vi "BN_outputLayer_with_FPGA.vi"(0 "Target_outX":fxp<+/-,32,8>[](array[numeric]), 1 "Out_hx":fxp<+/-,32,8>[](array[numeric]), 2 "Out_outX":fxp<+/-,32,8>[](array[numeric]), 3 "Learning rate":fxp<+/-,32,8>, 4 "Weights_outX_IN":fxp<+/-,32,8>[][](array[numeric])) -> (5 "Weights_outX_OUT":fxp<+/-,32,8>[][](array[numeric]))   [LabVIEW 2016]
uses:
  <vilib>/FPGAPlugInAG/myRIO-1900/niLvFpga_Open_myRIO-1900.vi
  <vilib>/rvi/interface/common/dynamic/niFpgaDynamicAddResources.vi
  <vilib>/Utility/error.llb/Error Cluster From Error Code.vi
  <vilib>/rvi/errors/niLvFpgaAdjustHostInterfaceError.vi
  <vilib>/FPGAPlugInAG/Dynamic/niLvFpga_Close_Dynamic.vi
  <vilib>/rvi/interface/nirviOpenFPGA/nirviOpenFPGA.xnode
  FPGA Bitfiles/Musicidentifier_FPGATarget_Update2layerWxFP_dcVOeM+zR40.lvbitx
  <vilib>/rvi/interface/nirviReadWriteControl/nirviReadWriteControl.xnode
  <vilib>/rvi/interface/nirviCloseFPGA/nirviCloseFPGA.xnode
  NiFpgaLv.dll
  <vilib>/rvi/interface/Simulation/niFpgaSimulationCallBeginRW.vi
panel:
  out "error out":errorcluster
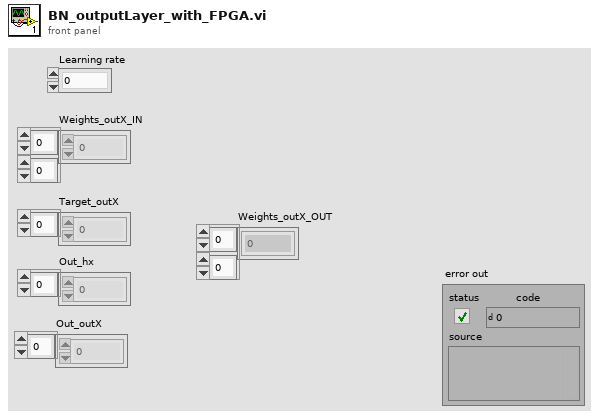
[diagram p1: front panel]
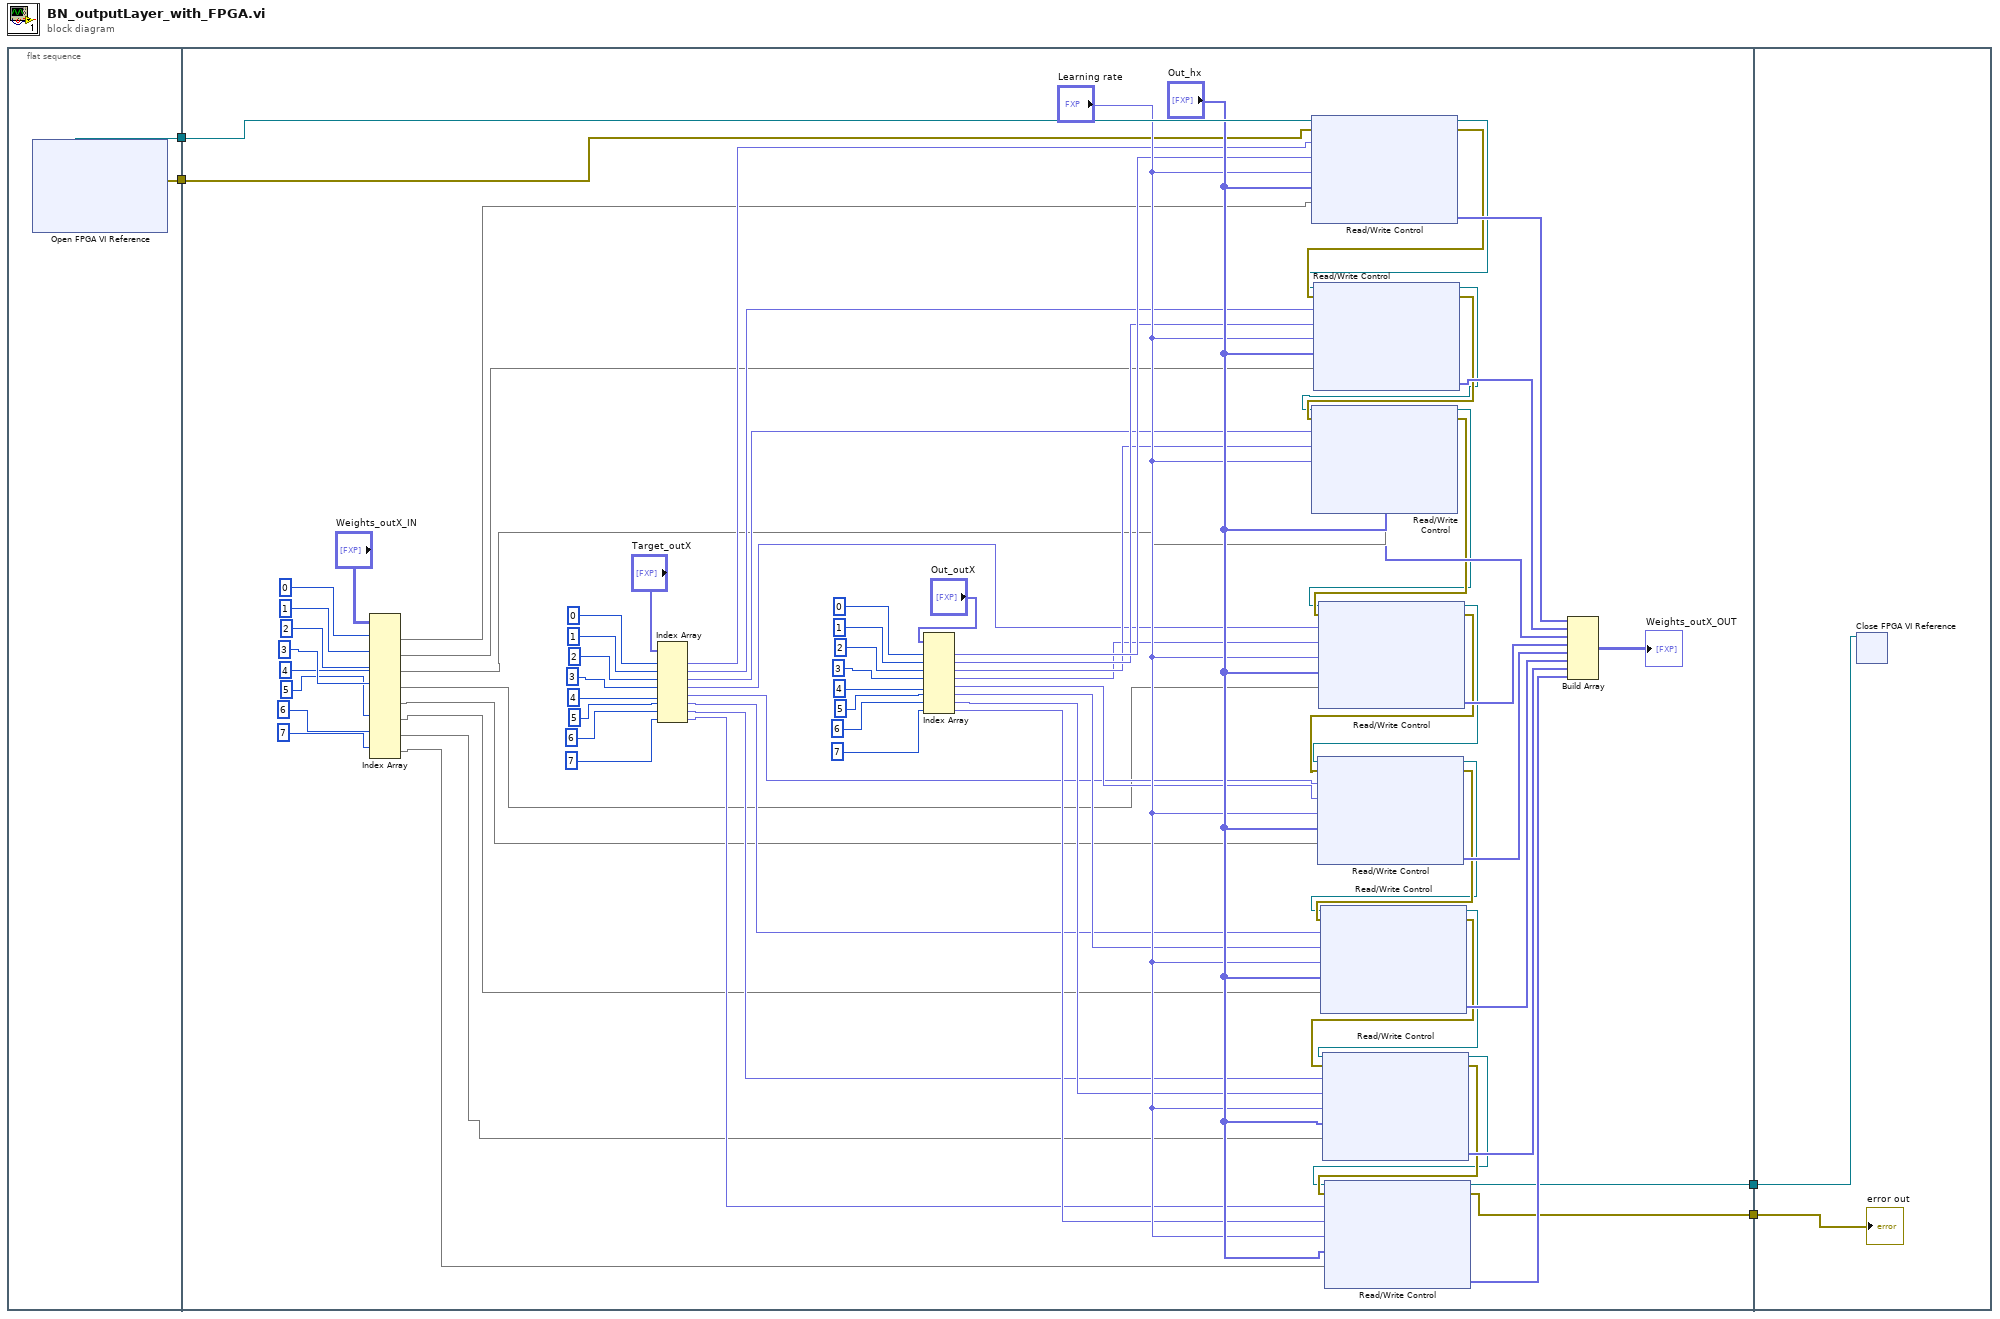
[diagram p0: block diagram]
diagram:
  n1 = flat-sequence {
    tunnel: [w6] -> w4
    tunnel: [w5] -> w3
    tunnel: w4 -> [w59]
    tunnel: w3 -> [w40]
    tunnel: [w7] -> w2
    tunnel: [w16] -> w1
    tunnel: w2 -> [w88]
    tunnel: w1 -> [w87]
    frame #0 {
      n2 = xnode "Open FPGA VI Reference"() -> ("FPGA VI Reference Out"=w6:refnum<k20>, "error out"=w5:errorcluster)  [unwired: 2 in]
    }
    frame #1 {
      n3 = Index Array(array="Weights_outX_IN", index (row) #1=0 ("index"), index (row) #2=1 ("index"), index (row) #3=2 ("index"), index (row) #4=3 ("index"), index (row) #5=4 ("index"), index (row) #6=5 ("index"), index (row) #7=6 ("index"), index (row) #8=7 ("index")) -> (element #1=w39:fxp<+/-,32,8>[], element #2=w38:fxp<+/-,32,8>[], element #3=w37:fxp<+/-,32,8>[], element #4=w36:fxp<+/-,32,8>[], element #5=w35:fxp<+/-,32,8>[], element #6=w34:fxp<+/-,32,8>[], element #7=w33:fxp<+/-,32,8>[], element #8=w32:fxp<+/-,32,8>[])  [unwired: 8 in]
      n4 = Index Array(array="Target_outX", index #1=0 ("index"), index #2=1 ("index"), index #3=2 ("index"), index #4=3 ("index"), index #5=4 ("index"), index #6=5 ("index"), index #7=6 ("index"), index #8=7 ("index")) -> (element #1=w48:fxp<+/-,32,8>, element #2=w47:fxp<+/-,32,8>, element #3=w46:fxp<+/-,32,8>, element #4=w45:fxp<+/-,32,8>, element #5=w44:fxp<+/-,32,8>, element #6=w43:fxp<+/-,32,8>, element #7=w42:fxp<+/-,32,8>, element #8=w41:fxp<+/-,32,8>)
      n5 = Index Array(array="Out_outX", index #1=0 ("index"), index #2=1 ("index"), index #3=2 ("index"), index #4=3 ("index"), index #5=4 ("index"), index #6=5 ("index"), index #7=6 ("index"), index #8=7 ("index")) -> (element #1=w56:fxp<+/-,32,8>, element #2=w55:fxp<+/-,32,8>, element #3=w54:fxp<+/-,32,8>, element #4=w53:fxp<+/-,32,8>, element #5=w52:fxp<+/-,32,8>, element #6=w51:fxp<+/-,32,8>, element #7=w50:fxp<+/-,32,8>, element #8=w49:fxp<+/-,32,8>)
      n6 = xnode "Read/Write Control"("FPGA VI Reference In"=w59, "error in"=w40, "Target_OutX"=w48, "2layer_OutX 2"=w56, "Learning rate"="Learning rate", "Array_Out_hx"="Out_hx", "Weights_2layer"=w39) -> ("FPGA VI Reference Out"=w14:refnum<k20>, "error out"=w22:errorcluster, "Weights_2layer_updated"=w31:fxp<+/-,32,8>[])
      n7 = xnode "Read/Write Control"("FPGA VI Reference In"=w14, "error in"=w22, "Target_OutX"=w47, "2layer_OutX 2"=w55, "Learning rate"="Learning rate", "Array_Out_hx"="Out_hx", "Weights_2layer"=w38) -> ("FPGA VI Reference Out"=w13:refnum<k20>, "error out"=w15:errorcluster, "Weights_2layer_updated"=w30:fxp<+/-,32,8>[])
      n8 = xnode "Read/Write Control"("FPGA VI Reference In"=w13, "error in"=w15, "Target_OutX"=w46, "2layer_OutX 2"=w54, "Learning rate"="Learning rate", "Array_Out_hx"="Out_hx", "Weights_2layer"=w37) -> ("FPGA VI Reference Out"=w12:refnum<k20>, "error out"=w21:errorcluster, "Weights_2layer_updated"=w29:fxp<+/-,32,8>[])
      n9 = xnode "Read/Write Control"("FPGA VI Reference In"=w12, "error in"=w21, "Target_OutX"=w45, "2layer_OutX 2"=w53, "Learning rate"="Learning rate", "Array_Out_hx"="Out_hx", "Weights_2layer"=w36) -> ("FPGA VI Reference Out"=w11:refnum<k20>, "error out"=w20:errorcluster, "Weights_2layer_updated"=w28:fxp<+/-,32,8>[])
      n10 = xnode "Read/Write Control"("FPGA VI Reference In"=w11, "error in"=w20, "Target_OutX"=w44, "2layer_OutX 2"=w52, "Learning rate"="Learning rate", "Array_Out_hx"="Out_hx", "Weights_2layer"=w35) -> ("FPGA VI Reference Out"=w10:refnum<k20>, "error out"=w19:errorcluster, "Weights_2layer_updated"=w27:fxp<+/-,32,8>[])
      n11 = xnode "Read/Write Control"("FPGA VI Reference In"=w10, "error in"=w19, "Target_OutX"=w43, "2layer_OutX 2"=w51, "Learning rate"="Learning rate", "Array_Out_hx"="Out_hx", "Weights_2layer"=w34) -> ("FPGA VI Reference Out"=w9:refnum<k20>, "error out"=w18:errorcluster, "Weights_2layer_updated"=w26:fxp<+/-,32,8>[])
      n12 = xnode "Read/Write Control"("FPGA VI Reference In"=w9, "error in"=w18, "Target_OutX"=w42, "2layer_OutX 2"=w50, "Learning rate"="Learning rate", "Array_Out_hx"="Out_hx", "Weights_2layer"=w33) -> ("FPGA VI Reference Out"=w8:refnum<k20>, "error out"=w17:errorcluster, "Weights_2layer_updated"=w25:fxp<+/-,32,8>[])
      n13 = xnode "Read/Write Control"("FPGA VI Reference In"=w8, "error in"=w17, "Target_OutX"=w41, "2layer_OutX 2"=w49, "Learning rate"="Learning rate", "Array_Out_hx"="Out_hx", "Weights_2layer"=w32) -> ("FPGA VI Reference Out"=w7:refnum<k20>, "error out"=w16:errorcluster, "Weights_2layer_updated"=w24:fxp<+/-,32,8>[])
      n14 = Build Array(w31, w30, w29, w28, w27, w26, w25, w24) -> (→"Weights_outX_OUT":fxp<+/-,32,8>[][])
    }
    frame #2 {
      n15 = xnode "Close FPGA VI Reference"("FPGA VI Reference In"=w88) -> ()  [unwired: 1 in, 1 out]
      "error out" <- w87
    }
  }
